vi "GetAlazar_SynthFoc - ATS-SDK.vi"(1 "Digitizer Settings":T4={"Digitizer delay (us) "=0.0, "rf points per line"=2048, "lines per plane"=128, "Samp Rate (Hz)"=100000000.0, "Additional dig delay (us)"=0.0, "Voltage Scale"=0.4, "Pre-Looks"=0, "Offset delay (us)"=0.0, "bits A/D"=8, "Avg Num"=1, "DigTimeOut"=5.0, "Rel Dig Delay"=0.0, "Dig Ch"=0, "LeCroyCluster"={"LeCroy Channels"=[TRUE, FALSE, FALSE, FALSE], "LC read pt offset"=0.0, "Sweep Avg"=FALSE}, "Main Digitizer"=enum."NI Digitizer", "Dig Config"=enum."Single channel", "Digitizer ID Cluster"={"Acqiris/Alazar/SP ID"=[], "NI Instr Handles"=[], "LeCroy VISA"="", "GaGe Handle"={"Handle"=0, "Sample size"=0, "Resolution"=0, "Offset"=0, "Channels"=0, "Boards"=0}, "ATS Ref"="ATS9350", "Acqiris Address"=["PCI::INSTR0"], "ADQRef"=refnum, "adq_cu_ptr"=refnum}, "Trigger Settings"={"Trig Source"=1, "Trig Coupling"=0, "Trig Slope"=0, "Level (mV)"=1500.0}, "Bulk Acq"=FALSE, "Bulk Start Indexes"=[], "Data Ref RF"=refnum, "NI ID/Channel"=[], "Total Dig CH"=1, "Xtra Ann Trig delay (us)"=10.0, "Fix Z Delay?"=FALSE, "One Way Transmission?"=FALSE, "Data Ref Log"=refnum} {"Trigger Settings"."Trig Slope" items=["Positive", "Negative"]; "Trigger Settings"."Level (mV)" format="%.2f"; "Trigger Settings"."Trig Coupling" items=["DC 1 MOhm", "AC 1 MOhm", "DC 50 Ohm", "AC 50 Ohm"]; "Trigger Settings"."Trig Source" items=["Chan 1", "External"]; "Rel Dig Delay" format="%.2f"; "DigTimeOut" format="%.2f"; "Avg Num" min=1; "Offset delay (us)" format="%.2f"; "Additional dig delay (us)" format="%.2f"; "Digitizer delay (us)" format="%.2f"}, 2 "AlazarCluster":T8, 4 "Reverse ?":bool, 5 "errorin":errorcluster, 6 "File Array":string[](array[string]), 7 "Ann Array Params":T1={"Synth Foc?"=FALSE, "Focal Zones"=41, "Switch T/R"=0, "Trans Geometry (mm)"={"Transducer"=0, "Geo Focus"=12.0, "a (radius)"=3.0, "# of rings"=5, "kerf space "=0.1, "Center Freq"=12.0}, "Sub Ap Excite?"=FALSE, "Full Array Scan?"=FALSE, "Xmt/Rcv"={"XMIT"=[TRUE, TRUE, TRUE, TRUE, TRUE], "RCV"=[TRUE, TRUE, TRUE, TRUE, TRUE]}, "PulseSpacing (us)"=0.0, "Xmit Ring"=0, "XMIT CHS"=0, "RCV CHS"=0, "GPU?"=FALSE, "Save TIFF?"=FALSE, "downfactor"=1, "RCV 1CH"=0} {"RCV 1CH" items=["All", "1", "2", "3", "4", "5"]; "Trans Geometry (mm)"."Transducer" items=["6D 12R 40 MHz"=0, "10D 31R 20 MHz"=1, "10D 23R 20 MHz"=2, "6D 23R 40 MHz"=3, "4.5D 10.7R 40 MHz"=4, "9D 23.5R 20 MHz"=5, "9D 25.8R 20MHz"=6, "Enter"=99]; "Switch T/R" min=1 max=5 step=1}, 8 "lines per plane":i32, 9 "Rcv Ring":i32) -> (12 "Gain Array":T10(array[cluster]), 13 "Raw VGain (scale)":dbl, 15 "VGain (dB)":dbl, 18 "Array out":i16[][][](array[numeric]), 19 "error out":errorcluster)   [LabVIEW 2022 SP3]
uses:
  -DigitizerRoutines/DigitizerSettings.ctl
  -DigitizerRoutines/Digitizer.ctl
  -DigitizerRoutines/DigConfig.ctl
  -DigitizerRoutines/DigitizerID.ctl
  C:/Windows/System32/ADQAPI_dotNet_helper.dll
  Annular Array/-AnnularRoutines/AnnularArray.ctl
  Annular Array/-AnnularRoutines/TransGeometry.ctl
  Annular Array/-AnnularRoutines/ArrayGeometry.ctl
  Annular Array/-SynthApperture/ProcImageHD_I16.vi
panel:
  out "Voltage Scale":T9
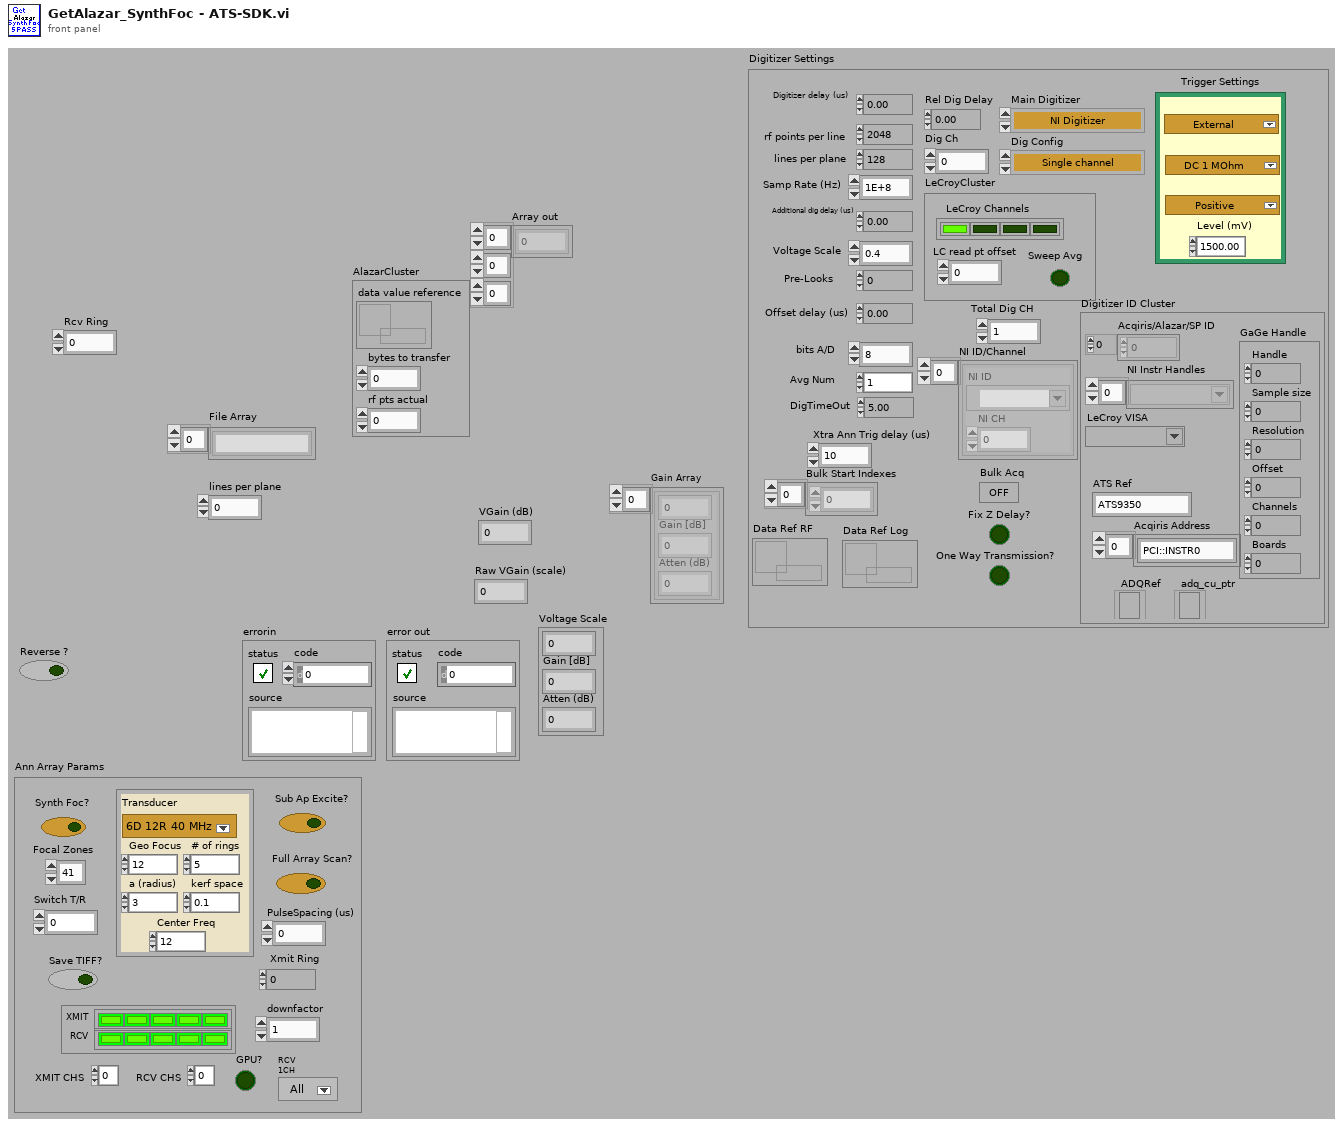
[diagram p1: front panel]
types:
  T1 = typedef "AnnularArray.ctl" = cluster{"Synth Foc?":bool, "Focal Zones":i16, "Switch T/R":i16, "Trans Geometry (mm)":T2, "Sub Ap Excite?":bool, "Full Array Scan?":bool, "Xmt/Rcv":cluster{"XMIT":bool[], "RCV":bool[]}, "PulseSpacing (us)":sgl, "Xmit Ring":i32, "XMIT CHS":u8, "RCV CHS":u8, "GPU?":bool, "Save TIFF?":bool, "downfactor":i32, "RCV 1CH":u16}
  T2 = typedef "TransGeometry.ctl" = cluster{"Transducer":T3, "Geo Focus":dbl, "a (radius)":dbl, "# of rings":i32, "kerf space ":dbl, "Center Freq":dbl}
  T3 = typedef "ArrayGeometry.ctl" = u16
  T4 = typedef "DigitizerSettings.ctl" = cluster{"Digitizer delay (us) ":dbl, "rf points per line":i32, "lines per plane":i32, "Samp Rate (Hz)":dbl, "Additional dig delay (us)":dbl, "Voltage Scale":dbl, "Pre-Looks":i32, "Offset delay (us)":dbl, "bits A/D":i8, "Avg Num":i32, "DigTimeOut":sgl, "Rel Dig Delay":sgl, "Dig Ch":i32, "LeCroyCluster":cluster{"LeCroy Channels":bool[], "LC read pt offset":dbl, "Sweep Avg":bool}, "Main Digitizer":T5, "Dig Config":T6, "Digitizer ID Cluster":T7, "Trigger Settings":cluster{"Trig Source":u16, "Trig Coupling":u16, "Trig Slope":u16, "Level (mV)":dbl}, "Bulk Acq":bool, "Bulk Start Indexes":i32[], "Data Ref RF":refnum<data-value>, "NI ID/Channel":cluster{"NI ID":refnum<k15>, "NI CH":i32}[], "Total Dig CH":i32, "Xtra Ann Trig delay (us)":dbl, "Fix Z Delay?":bool, "One Way Transmission?":bool, "Data Ref Log":refnum<data-value>}
  T5 = typedef "Digitizer.ctl" = enum16{"Acqiris Digitizer", "NI Digitizer", "LeCroy", "GaGe", "AlazarTech", "No Digitizer", "Teledyne"}
  T6 = typedef "DigConfig.ctl" = enum16{"Single channel", "2 Chans w/ 2 Acqiris", "2 Chans w/ 1 Acqiris", "5-CH Pulser New", "5-CH pulser w/ ann array", "5-pass style ann array", "Empty"}
  T7 = typedef "DigitizerID.ctl" = cluster{"Acqiris/Alazar/SP ID":u32[], "NI Instr Handles":refnum<k15>[], "LeCroy VISA":refnum<visa-resource-name>, "GaGe Handle":cluster{"Handle":u32, "Sample size":u32, "Resolution":i32, "Offset":i32, "Channels":u32, "Boards":u32}, "ATS Ref":string, "Acqiris Address":string[], "ADQRef":refnum<k24>, "adq_cu_ptr":refnum<k24>}
  T8 = cluster{"data value reference":refnum<data-value>, "bytes to transfer":u32, "rf pts actual":u32}
  T9 = cluster{sgl, "Gain [dB]  ":sgl, "Atten (dB)":sgl}
  T10 = cluster{sgl, "Gain [dB]  ":sgl, "Atten (dB)":sgl}[]
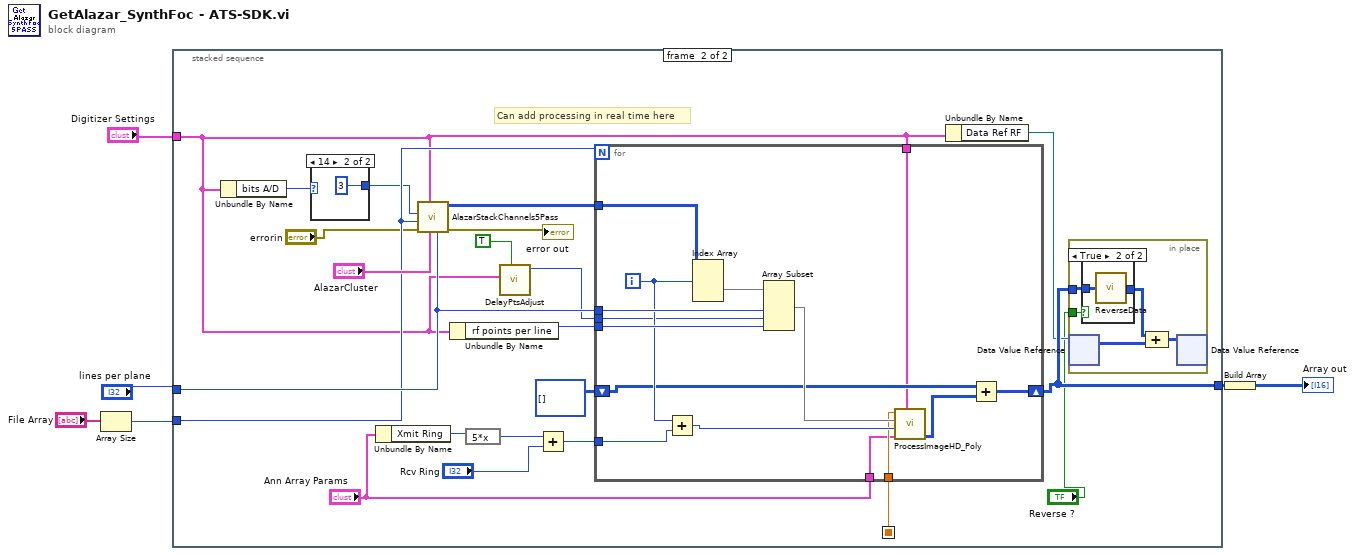
[diagram p0: block diagram]
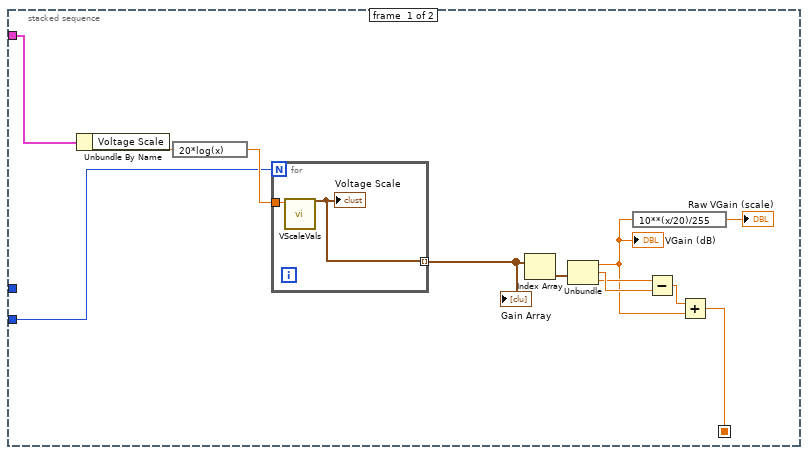
[diagram p2: hidden frame]
diagram:
  n1 = Array Size(array="File Array") -> (size(s)=w1:i32)
  n2 = stacked-sequence {
    seq-local: [w10 _] -> [_ w28]
    tunnel: "lines per plane" -> [_ w31]
    tunnel: w1 -> [w9 w30]
    tunnel: [_ w36] -> w4
    tunnel: "Digitizer Settings" -> [w8 w23]
    frame #0 {
      n3 = Unbundle By Name(w8) -> ("Voltage Scale"=w7:dbl)
      n4 = expression code="20*log(x)"(w7) -> (w14:dbl)
      n5 = for {
        N: w9 -> [_]
        tunnel: [w19] -> w11 mode=indexing
        tunnel: w14 -> [w20]
        n6 = call "VScaleVals.vi"("Full Scale"=w20) -> ("Voltage Scale"=w19:T9)  [unwired: 8 in, 2 out]
        "Voltage Scale" <- w19
      }
      "Gain Array" <- w11
      n7 = Index Array(array=w11) -> (element=w13:T9)  [unwired: 1 in]
      n8 = Unbundle(w13) -> (w16:sgl, "Gain [dB]"=w18:sgl, "Atten (dB)"=w17:sgl)
      "VGain (dB)" <- w16
      n9 = expression code="10**(x/20)/255"(w16) -> (→"Raw VGain (scale)":sgl)
      n10 = Subtract(x=w17, y=w18) -> (x-y=w15:sgl)
      n11 = Add(x=w15, y=w16) -> (x+y=w10:sgl)
    }
    frame #1 {
      # "Can add processing in real time here"
      n12 = Unbundle By Name(w23) -> ("bits A/D"=w25:i8)
      n13 = case shown="14" w25 {
        tunnel: [_ u16 3 ("Extra Shift")] -> w27
        frame 0, Default {
        }
        frame 14 {
        }
      }
      n14 = Unbundle By Name("Ann Array Params") -> ("Xmit Ring"=w38:i32)
      n15 = call "AlazarStackChannels5Pass.vi"("lines per plane"=w31, "AlazarCluster"="AlazarCluster", "Digitizer Settings"=w23, "error in"="errorin", "Channels"=w30, "Extra Shift"=w27) -> ("error out"=→"error out":errorcluster, "ChStackDataOut"=w33:i16[][][])  [unwired: 2 in, 2 out]
      n16 = Unbundle By Name(w23) -> ("rf points per line"=w24:i32)
      n17 = expression code="5*x"(w38) -> (w42:i32)
      n18 = call "DelayPtsAdjust.vi"("CalcPt?"=TRUE, "Digitizer Settings"=w23) -> ("PostDelayCorrection"=w22:u32)  [unwired: 8 in, 1 out]
      n19 = Add(x=w42, y="Rcv Ring") -> (x+y=w40:i32)
      n20 = for {
        N: w30 -> [_]
        tunnel: w33 -> [w66]
        tunnel: w24 -> [w65]
        tunnel: w31 -> [w64]
        tunnel: w40 -> [w61]
        tunnel: w28 -> [w58]
        shift-right: [w56] -> w36
        shift-left: i16[][] [] -> [w55]
        tunnel: w23 -> [w54]
        tunnel: "Ann Array Params" -> [w53]
        tunnel: w22 -> [w52]
        i -> [w62]
        n21 = Add(x=w62, y=w61) -> (x+y=w60:i32)
        n22 = Index Array(array=w66, index (dim 0)=w62) -> (element=w63:i16[][])  [unwired: 2 in]
        n23 = Array Subset(array=w63, length (row)=w64, index (col)=w52, length (col)=w65) -> (w59:i16[][])  [unwired: 1 in]
        n24 = call-poly "ProcessImageHD_Poly.vi"("Digitizer Settings"=w54, "Ann Array Params"=w53, "T/R Ring"=w60, "Scan Data In"=w59, "Att (dB)"=w58) -> ("Synth App Out"=w57:i16[][])  [unwired: 3 in, 1 out]
        n25 = Add(x=w55, y=w57) -> (x+y=w56:i16[][])
      }
      n26 = Unbundle By Name(w23) -> ("Data Ref RF"=w35:refnum<data-value>)
      n27 = in-place {
        in-place-border: w36 -> [w45]
        in-place-border: "Reverse ?" -> [w44]
        n28 = in-place-dvr #1(w35) -> (w48:i16[][])  [unwired: 1 out]
        n29 = case shown="True" w44 {
          tunnel: w45 -> [w49 w51]
          tunnel: [w49 w50] -> w46
          frame False {
          }
          frame True {
            n30 = call "ReverseData.vi"("Array in"=w51) -> ("Array out"=w50:i16[][])
          }
        }
        n31 = Compound Arithmetic op=ADD(w46, w48) -> (w47:i16[][])
        n32 = in-place-dvr #1(w47) -> ()  [unwired: 2 out]
      }
    }
  }
  n33 = Build Array(w4) -> (→"Array out":i16[][][])
